vi "Aircraft Attitude.vi"   [LabVIEW 2014]
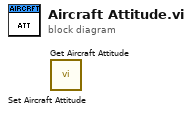
[diagram p0: block diagram]
diagram:
  n1 = call "Set Aircraft Attitude.vi"() -> ()  [unwired: 10 in, 2 out]
  n2 = call "Get Aircraft Attitude.vi"() -> ()  [unwired: 10 in, 2 out]
